vi "Test WhileLoop Iterator Info.vi"() -> ()   [LabVIEW 2018]
panel:
  out "Class Name":string
  in  "vi path":path=path "C:/Users/lubo/Documents/LabView/LabVIEW-Universal-Transcriptor/Test/Examples For Parsing/Example WhileLoop ForLoop.vi"
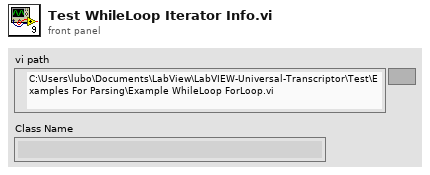
[diagram p1: front panel]
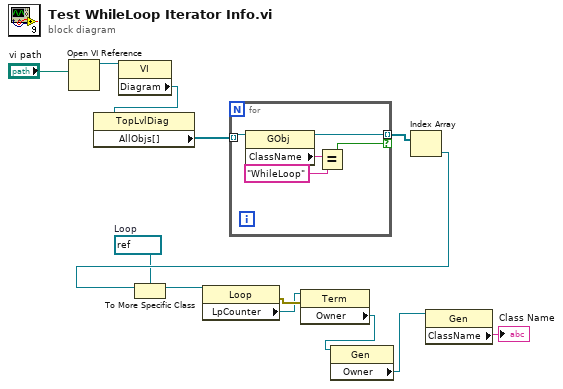
[diagram p0: block diagram]
diagram:
  w6 = refnum<vi> refnum  # Loop
  n1 = Open VI Reference(vi path="vi path") -> (vi reference=w12:refnum<vi>)  [unwired: 5 in, 1 out]
  n2 = property class="VI"(reference=w12) -> ("Diagram"=w11:refnum<vi>)  [unwired: 1 in, 2 out]
  n3 = property class="TopLvlDiag"(reference=w11) -> ("AllObjs[]"=w10:refnum<vi>[])  [unwired: 1 in, 2 out]
  n4 = for {
    tunnel: w10 -> [w18] mode=indexing
    tunnel: [w15] -> w9 mode=indexing if=w14
    n5 = property class="GObj"(reference=w18) -> (reference out=w15:refnum<vi>, "ClassName"=w17:string)  [unwired: 1 in, 1 out]
    n6 = Equal?(x=w17, y="WhileLoop") -> (x = y?=w14:bool)
  }
  n7 = Index Array(array=w9) -> (element=w8:refnum<vi>)  [unwired: 1 in]
  n8 = To More Specific Class(target class=w6, reference=w8) -> (specific class reference=w7:refnum<vi>)  [unwired: 1 in, 1 out]
  n9 = property class="Loop"(reference=w7) -> (error out=w5:errorcluster, "LpCounter"=w4:refnum<vi>)  [unwired: 1 in, 1 out]
  n10 = property class="Term"(reference=w4, error in=w5) -> ("Owner"=w2:refnum<vi>)  [unwired: 2 out]
  n11 = property class="Gen"(reference=w2) -> ("Owner"=w1:refnum<vi>)  [unwired: 1 in, 2 out]
  n12 = property class="Gen"(reference=w1) -> ("ClassName"=→"Class Name":string)  [unwired: 1 in, 2 out]
